vi "CRYRub & Buzz Pp[k].vi"(8 "Pe[k]":dbl[](array[numeric]), 9 "Version":i32, 10 "Real matrix":dbl[][](array[numeric])) -> (3 "Pp[k]":dbl[](array[numeric]))   [LabVIEW 2013]
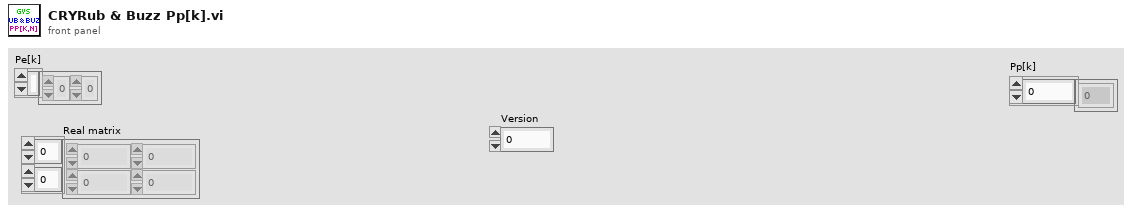
[diagram p1: front panel]
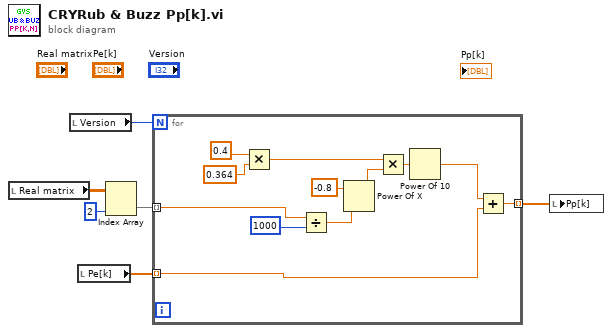
[diagram p0: block diagram]
diagram:
  n1 = local read "Real matrix"() -> (w4:dbl[][])
  n2 = local read "Version"() -> (w6:i32)
  n3 = local read "Pe[k]"() -> (w2:dbl[])
  n4 = Index Array(array=w4, index (col)=2) -> (element=w3:dbl[])  [unwired: 1 in]
  n5 = for {
    N: w6 -> [_]
    tunnel: w3 -> [w10] mode=indexing
    tunnel: [w8] -> w1 mode=indexing
    tunnel: w2 -> [w7] mode=indexing
    n6 = Multiply(x=0.4, y=0.364) -> (x*y=w13:dbl)
    n7 = Divide(x=w10, y=1000) -> (x/y=w16:dbl)
    n8 = Power Of X ("Power Of X.vi")(1:w16, 2:-0.8) -> (0:w14:dbl)
    n9 = Multiply ("Multiply.vi")(x=w13, y=w14) -> (x*y=w12:dbl)
    n10 = Power Of 10(x=w12) -> (10^x=w9:dbl)
    n11 = Add ("Add.vi")(x=w9, y=w7) -> (x+y=w8:dbl)
  }
  n12 = local write "Pp[k]"(w1) -> ()
